vi "Results_Column_Types.vi"() -> (1 "Correlation":string, 2 "Metadata":string, 3 "Instrument":string)   [LabVIEW 2022 SP3]
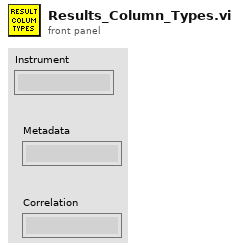
[diagram p1: front panel]
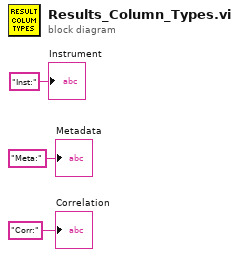
[diagram p0: block diagram]
diagram:
  "Instrument" <- "Inst:" ("Instrument")
  "Metadata" <- "Meta:" ("Metadata")
  "Correlation" <- "Corr:" ("Correlation")
